vi "Read Behavior.vi"(8 "error in (no error)":errorcluster, 11 "Attribute.StartupBehavior in":refnum<class "Attribute.StartupBehavior.lvclass">) -> (0 "error out":errorcluster, 2 "Behavior":T1, 3 "Attribute.StartupBehavior out":refnum<class "Attribute.StartupBehavior.lvclass">)   [LabVIEW 2021, in "smo.lvlib" / "Attribute.StartupBehavior.lvclass"]
uses:
  Attribute.StartupBehavior.lvclass
  Attribute.StartupBehavior.lvclass/Attribute.StartupBehavior.ctl
  ProcessStartupBehavior.ctl
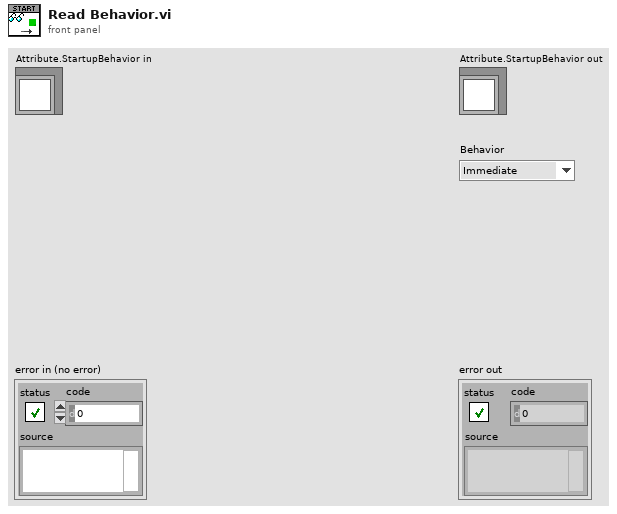
[diagram p1: front panel]
types:
  T1 = typedef "smo.lvlib/Attribute.StartupBehavior.lvclass/ProcessStartupBehavior.ctl" = enum16{"Immediate", "First Call", "Never"}
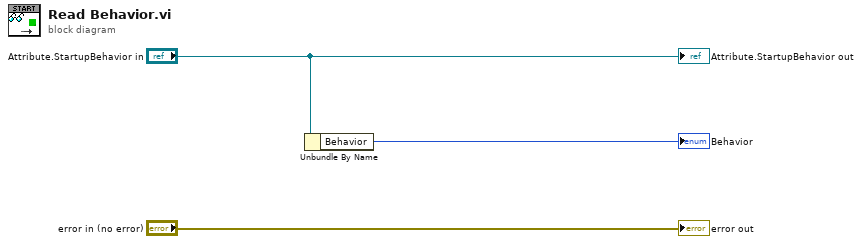
[diagram p0: block diagram]
diagram:
  n1 = Unbundle By Name("Attribute.StartupBehavior in") -> ("Behavior"=→"Behavior":T1)
  "error out" <- "error in (no error)"
  "Attribute.StartupBehavior out" <- "Attribute.StartupBehavior in"
